vi "DAQInit.vi"(4 "AOStartTrigger":tag="/DAQ_6110/ao/StartTrigger", 5 "AIStartTrigger":tag="/DAQ_6110/ai/StartTrigger", 6 "Scan/Meas Parameters":T5={"Pixel Dwell Time (s)"=0.0001, "Pixel Size"=200.0, "X Min (V)"=-7.5, "X Max (V)"=7.5, "Y Min (V)"=-7.5, "Y Max (V)"=7.5, "XY Factor (1/V)"=0.2}, 7 "Calibration Parameters":T4={"Target Lifetime (s)"=4e-09, "Integration Time (s)"=0.1, "Calibration Steps"=500.0}, 8 "error in":errorcluster, 9 "Functions":T6(ring)=enum."Measurement", 10 "Global Parameters":T1={"DC AI Min (V)"=0.0015, "DC AI Max (V)"=0.06, "Mixer AI Min (V)"=-0.3, "Mixer AI Max (V)"=0.3, "Bias AO Min (V)"=-1.0, "Bias AO Max (V)"=7.0, "Scan AO Min (V)"=-10.0, "Scan AO Max (V)"=10.0, "Fast Samp Freq (Hz)"=2500000.0, "Slow Samp Freq (Hz)"=250000.0}, 11 "DAQ Channels":T3) -> (0 "error out":errorcluster, 2 "Expected Time (s)":dbl=98.154, 3 "Tasks Out":T2)   [LabVIEW 2018]
uses:
  <vilib>/DAQmx/create/channels.llb/DAQmx Create Channel (AO-Voltage-Basic).vi
  <vilib>/DAQmx/configure/timing.llb/DAQmx Timing (Sample Clock).vi
  <vilib>/DAQmx/create/channels.llb/DAQmx Create Channel (AI-Voltage-Basic).vi
  <vilib>/DAQmx/configure/trigger.llb/DAQmx Start Trigger (Digital Edge).vi
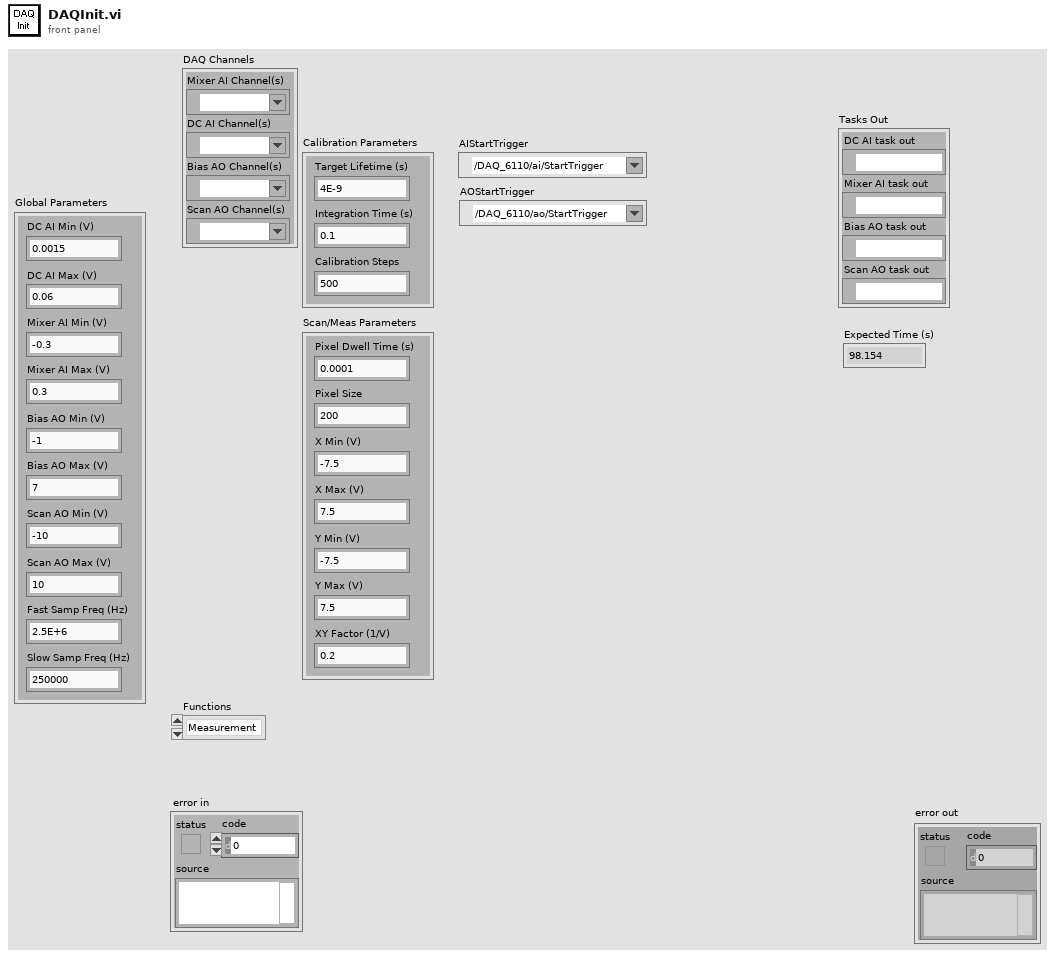
[diagram p1: front panel]
types:
  T1 = cluster{"DC AI Min (V)":dbl, "DC AI Max (V)":dbl, "Mixer AI Min (V)":dbl, "Mixer AI Max (V)":dbl, "Bias AO Min (V)":dbl, "Bias AO Max (V)":dbl, "Scan AO Min (V)":dbl, "Scan AO Max (V)":dbl, "Fast Samp Freq (Hz)":dbl, "Slow Samp Freq (Hz)":dbl}
  T2 = cluster{"DC AI task out":refnum<k21>, "Mixer AI task out":refnum<k21>, "Bias AO task out":refnum<k21>, "Scan AO task out":refnum<k21>}
  T3 = cluster{"Mixer AI Channel(s)":tag, "DC AI Channel(s)":tag, "Bias AO Channel(s) ":tag, "Scan AO Channel(s)":tag}
  T4 = cluster{"Target Lifetime (s)":dbl, "Integration Time (s)":dbl, "Calibration Steps":dbl}
  T5 = cluster{"Pixel Dwell Time (s)":dbl, "Pixel Size":dbl, "X Min (V)":dbl, "X Max (V)":dbl, "Y Min (V)":dbl, "Y Max (V)":dbl, "XY Factor (1/V)":dbl}
  T6 = enum32{"Calibration", "Fast Scan", "Measurement"}
  T7 = cluster{"task out":refnum<k21>, "task out":refnum<k21>, "task out":refnum<k21>, "task out":refnum<k21>}
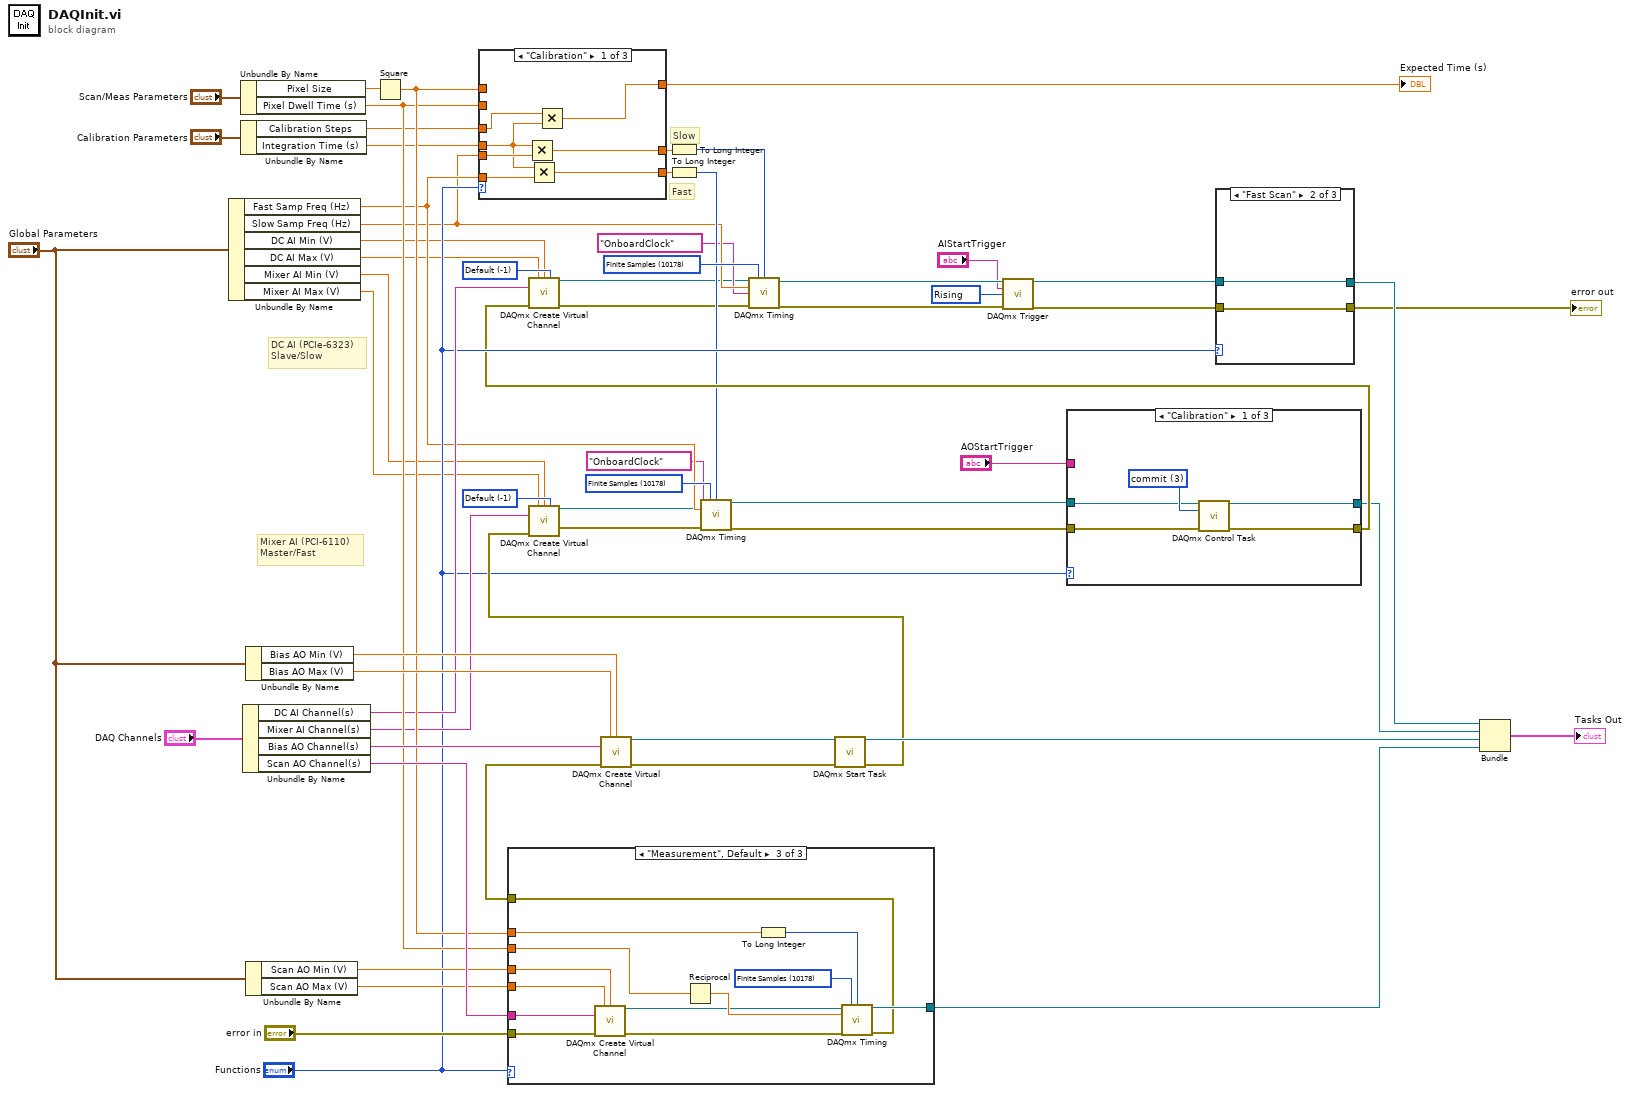
[diagram p0: block diagram]
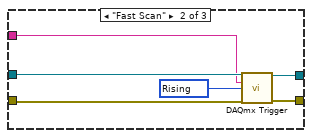
[diagram p2: hidden frame]
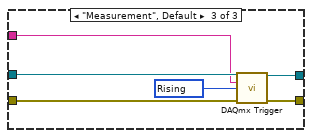
[diagram p3: hidden frame]
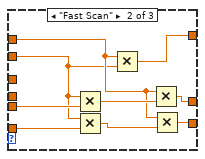
[diagram p4: hidden frame]
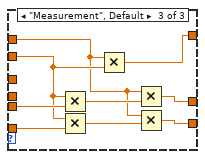
[diagram p5: hidden frame]
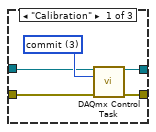
[diagram p6: hidden frame]
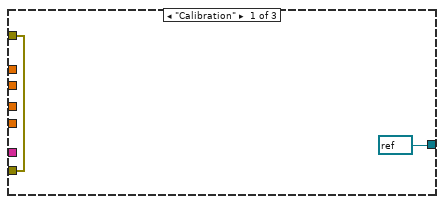
[diagram p8: hidden frame]
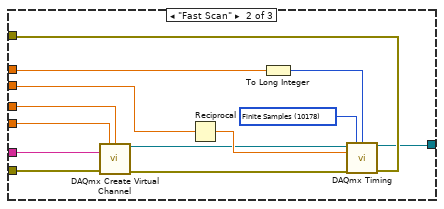
[diagram p9: hidden frame]
diagram:
  w14 = 10280 items=["Rising"=10280, "Falling"=10171] ("edge")
  w35 = 10178 items=["Finite Samples"=10178, "Continuous Samples"=10123, "Hardware Timed Single Point"=12522] ("sample mode")
  w36 = -1 items=["Default"=-1, "RSE"=10083, "NRSE"=10078, "Differential"=10106, "Pseudodifferential"=12529] ("input terminal configuration")
  w44 = 10178 items=["Finite Samples"=10178, "Continuous Samples"=10123, "Hardware Timed Single Point"=12522] ("sample mode")
  w45 = -1 items=["Default"=-1, "RSE"=10083, "NRSE"=10078, "Differential"=10106, "Pseudodifferential"=12529] ("input terminal configuration")
  # "Fast"
  # "Slow"
  # "DC AI (PCIe-6323)\nSlave/Slow"
  # "Mixer AI (PCI-6110)\nMaster/Fast"
  n1 = Unbundle By Name("Global Parameters") -> ("Fast Samp Freq (Hz)"=w25:dbl, "Slow Samp Freq (Hz)"=w21:dbl, "DC AI Min (V)"=w6:dbl, "DC AI Max (V)"=w4:dbl, "Mixer AI Min (V)"=w5:dbl, "Mixer AI Max (V)"=w3:dbl)
  n2 = Unbundle By Name("Scan/Meas Parameters") -> ("Pixel Size"=w54:dbl, "Pixel Dwell Time (s)"=w42:dbl)
  n3 = Unbundle By Name("Calibration Parameters") -> ("Calibration Steps"=w38:dbl, "Integration Time (s)"=w40:dbl)
  n4 = Unbundle By Name("DAQ Channels") -> ("DC AI Channel(s)"=w32:tag, "Mixer AI Channel(s)"=w33:tag, "Bias AO Channel(s)"=w49:tag, "Scan AO Channel(s)"=w57:tag)
  n5 = Unbundle By Name("Global Parameters") -> ("Bias AO Min (V)"=w47:dbl, "Bias AO Max (V)"=w48:dbl)
  n6 = Unbundle By Name("Global Parameters") -> ("Scan AO Min (V)"=w55:dbl, "Scan AO Max (V)"=w56:dbl)
  n7 = Square(x=w54) -> (x^2=w43:dbl)
  n8 = case shown="\"Calibration\"" "Functions" {
    tunnel: w21 -> [w67 w71 w84]
    tunnel: w43 -> [_ w72 w77]
    tunnel: w42 -> [_ w69 w80]
    tunnel: [w66 w75 w83] -> w41
    tunnel: w40 -> [w63 _ _]
    tunnel: [w64 w74 w82] -> w39
    tunnel: w38 -> [w65 _ _]
    tunnel: w25 -> [w62 w70 w81]
    tunnel: [w61 w73 w79] -> w27
    frame "Calibration" {
      n9 = Multiply(x=w63, y=w67) -> (x*y=w66:dbl)
      n10 = Multiply(x=w63, y=w62) -> (x*y=w61:dbl)
      n11 = Multiply(x=w65, y=w63) -> (x*y=w64:dbl)
    }
    frame "Fast Scan" {
      n12 = Multiply(x=w69, y=w71) -> (x*y=w76:dbl)
      n13 = Multiply(x=w69, y=w70) -> (x*y=w68:dbl)
      n14 = Multiply(x=w72, y=w69) -> (x*y=w74:dbl)
      n15 = Multiply(x=w72, y=w76) -> (x*y=w75:dbl)
      n16 = Multiply(x=w72, y=w68) -> (x*y=w73:dbl)
    }
    frame "Measurement", Default {
      n17 = Multiply(x=w80, y=w84) -> (x*y=w85:dbl)
      n18 = Multiply(x=w80, y=w81) -> (x*y=w78:dbl)
      n19 = Multiply(x=w77, y=w80) -> (x*y=w82:dbl)
      n20 = Multiply(x=w77, y=w85) -> (x*y=w83:dbl)
      n21 = Multiply(x=w77, y=w78) -> (x*y=w79:dbl)
    }
  }
  "Expected Time (s)" <- w39
  n22 = case shown="\"Measurement\", Default" "Functions" {
    tunnel: "error in" -> [w87 w89 w113]
    tunnel: w57 -> [_ w90 w112]
    tunnel: w56 -> [_ w91 w111]
    tunnel: w55 -> [_ w92 w110]
    tunnel: w42 -> [_ w93 w104]
    tunnel: w43 -> [_ w94 w103]
    tunnel: [refnum<k21> refnum ("task out") w88 w102] -> w53
    tunnel: [w87 w95 w101] -> w50
    frame "Calibration" {
    }
    frame "Fast Scan" {
      w100 = 10178 items=["Finite Samples"=10178, "Continuous Samples"=10123, "Hardware Timed Single Point"=12522] ("sample mode")
      n23 = call-poly <vilib>:"DAQmx Create Virtual Channel.vi"("maximum value"=w91, "minimum value"=w92, "physical channels"=w90, "error in"=w89) -> ("task out"=w97:refnum<k21>, "error out"=w96:errorcluster)  [unwired: 10 in]
      n24 = Reciprocal(x=w93) -> (1/x=w99:dbl)
      n25 = To Long Integer(number=w94) -> (32bit integer=w98:i32)
      n26 = call-poly <vilib>:"DAQmx Timing.vi"("task/channels in"=w97, "sample mode"=w100, "samples per channel"=w98, "rate"=w99, "error in"=w96) -> ("task out"=w88:refnum<k21>, "error out"=w95:errorcluster)  [unwired: 9 in]
    }
    frame "Measurement", Default {
      w109 = 10178 items=["Finite Samples"=10178, "Continuous Samples"=10123, "Hardware Timed Single Point"=12522] ("sample mode")
      n27 = call-poly <vilib>:"DAQmx Create Virtual Channel.vi"("maximum value"=w111, "minimum value"=w110, "physical channels"=w112, "error in"=w113) -> ("task out"=w106:refnum<k21>, "error out"=w105:errorcluster)  [unwired: 10 in]
      n28 = Reciprocal(x=w104) -> (1/x=w108:dbl)
      n29 = To Long Integer(number=w103) -> (32bit integer=w107:i32)
      n30 = call-poly <vilib>:"DAQmx Timing.vi"("task/channels in"=w106, "sample mode"=w109, "samples per channel"=w107, "rate"=w108, "error in"=w105) -> ("task out"=w102:refnum<k21>, "error out"=w101:errorcluster)  [unwired: 9 in]
    }
  }
  n31 = call-poly <vilib>:"DAQmx Create Virtual Channel.vi"("maximum value"=w48, "minimum value"=w47, "physical channels"=w49, "error in"=w50) -> ("task out"=w52:refnum<k21>, "error out"=w51:errorcluster)  [unwired: 10 in]
  n32 = To Long Integer(number=w41) -> (32bit integer=w30:i32)
  n33 = To Long Integer(number=w27) -> (32bit integer=w26:i32)
  n34 = call <vilib>:"DAQmx Start Task.vi"("task/channels in"=w52, "error in"=w51) -> ("task out"=w46:refnum<k21>, "error out"=w34:errorcluster)  [unwired: 12 in]
  n35 = call-poly <vilib>:"DAQmx Create Virtual Channel.vi"("maximum value"=w3, "minimum value"=w5, "input terminal configuration"=w36, "physical channels"=w33, "error in"=w34) -> ("task out"=w24:refnum<k21>, "error out"=w23:errorcluster)  [unwired: 9 in]
  n36 = call-poly <vilib>:"DAQmx Timing.vi"("task/channels in"=w24, "sample mode"=w35, "samples per channel"=w26, "rate"=w25, "source"=tag "OnboardClock", "error in"=w23) -> ("task out"=w18:refnum<k21>, "error out"=w17:errorcluster)  [unwired: 8 in]
  n37 = case shown="\"Calibration\"" "Functions" {
    tunnel: w17 -> [w116 w122 w129]
    tunnel: w18 -> [w117 w123 w128]
    tunnel: [w115 w121 w127] -> w29
    tunnel: [w114 w120 w126] -> w22
    tunnel: "AOStartTrigger" -> [_ w119 w125]
    frame "Calibration" {
      w118 = 3 items=["verify"=2, "reserve"=4, "commit"=3, "unreserve"=5, "abort"=6] ("action")
      n38 = call <vilib>:"DAQmx Control Task.vi"("task/channels in"=w117, "action"=w118, "error in"=w116) -> ("task out"=w114:refnum<k21>, "error out"=w115:errorcluster)  [unwired: 11 in]
    }
    frame "Fast Scan" {
      w124 = 10280 items=["Rising"=10280, "Falling"=10171] ("edge")
      n39 = call-poly <vilib>:"DAQmx Trigger.vi"("task/channels in"=w123, "source"=w119, "edge"=w124, "error in"=w122) -> ("task out"=w120:refnum<k21>, "error out"=w121:errorcluster)  [unwired: 10 in]
    }
    frame "Measurement", Default {
      w130 = 10280 items=["Rising"=10280, "Falling"=10171] ("edge")
      n40 = call-poly <vilib>:"DAQmx Trigger.vi"("task/channels in"=w128, "source"=w125, "edge"=w130, "error in"=w129) -> ("task out"=w126:refnum<k21>, "error out"=w127:errorcluster)  [unwired: 10 in]
    }
  }
  n41 = call-poly <vilib>:"DAQmx Create Virtual Channel.vi"("maximum value"=w4, "minimum value"=w6, "input terminal configuration"=w45, "physical channels"=w32, "error in"=w29) -> ("task out"=w16:refnum<k21>, "error out"=w15:errorcluster)  [unwired: 9 in]
  n42 = call-poly <vilib>:"DAQmx Timing.vi"("task/channels in"=w16, "sample mode"=w44, "samples per channel"=w30, "rate"=w21, "source"=tag "OnboardClock", "error in"=w15) -> ("task out"=w11:refnum<k21>, "error out"=w8:errorcluster)  [unwired: 8 in]
  n43 = call-poly <vilib>:"DAQmx Trigger.vi"("task/channels in"=w11, "source"="AIStartTrigger", "edge"=w14, "error in"=w8) -> ("task out"=w10:refnum<k21>, "error out"=w9:errorcluster)  [unwired: 10 in]
  n44 = case shown="\"Fast Scan\"" "Functions" {
    tunnel: w9 -> [w133 w136 w138]
    tunnel: w10 -> [w134 w137 w139]
    tunnel: [w132 w136 w138] -> w12
    tunnel: [w131 w137 w139] -> w13
    frame "Calibration" {
      w135 = 3 items=["verify"=2, "reserve"=4, "commit"=3, "unreserve"=5, "abort"=6] ("action")
      n45 = call <vilib>:"DAQmx Control Task.vi"("task/channels in"=w134, "action"=w135, "error in"=w133) -> ("task out"=w131:refnum<k21>, "error out"=w132:errorcluster)  [unwired: 11 in]
    }
    frame "Fast Scan" {
    }
    frame "Measurement", Default {
    }
  }
  "error out" <- w12
  n46 = Bundle("task out"=w13, "task out"=w22, "task out"=w46, "task out"=w53) -> (→"Tasks Out":T7)  [unwired: 1 in]
